vi "NI VeriStand - Get Raw Value.vi"(8 "error in":errorcluster, 10 "Channel Name":string, 11 "Calibration In":T1) -> (0 "error out":errorcluster, 2 "Value":dbl, 3 "Calibration Out":T1)   [LabVIEW 2020, in "NI_VS Calibration ExecutionAPI.lvlib"]
doc: "Returns the value the specified channel measures or generates before NI VeriStand applies any calibration or scaling."
uses:
  <vilib>/NI VeriStand/Execution/Calibration/NI_VS Calibration ExecutionAPI.lvlib
  <vilib>/NI VeriStand/Execution/Calibration/CalibrationAPI.ctl
  NationalInstruments.VeriStand.ClientAPI
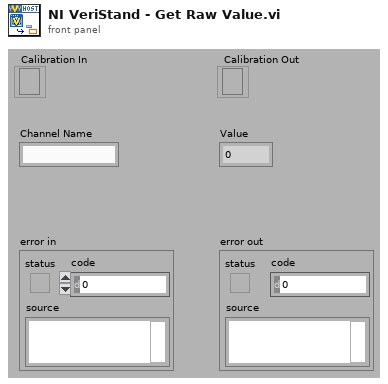
[diagram p1: front panel]
types:
  T1 = typedef "NI_VS Calibration ExecutionAPI.lvlib/CalibrationAPI.ctl" = refnum<k24>
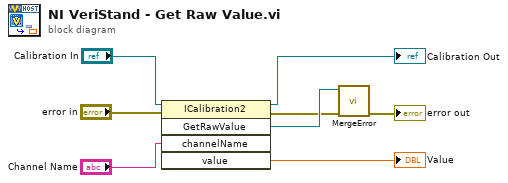
[diagram p0: block diagram]
diagram:
  n1 = invoke class="ICalibration2" method="GetRawValue"(reference="Calibration In", error in="error in", "channelName"="Channel Name") -> (reference out=→"Calibration Out":T1, error out=w1:errorcluster, "GetRawValue"=w8:refnum<k24>, "value"=→"Value":dbl)  [unwired: 2 in, 1 out]
  n2 = call <vilib>:"MergeError.vi"("error in (no error)"=w1, "Error"=w8) -> ("error out"=→"error out":errorcluster)  [unwired: 9 out]
